vi "Initialize.vi"(8 "error in (no error)":errorcluster, 11 "DemoStepMotor in":refnum<class "DemoStepMotor.lvclass">) -> (0 "error out":errorcluster, 3 "DemoStepMotor out":refnum<class "DemoStepMotor.lvclass">)   [LabVIEW 2020, in "DemoStepMotor.lvlib" / "DemoStepMotor.lvclass"]
uses:
  DemoStepMotor.lvclass
  <vilib>/ActorFramework/Actor/Actor.lvclass
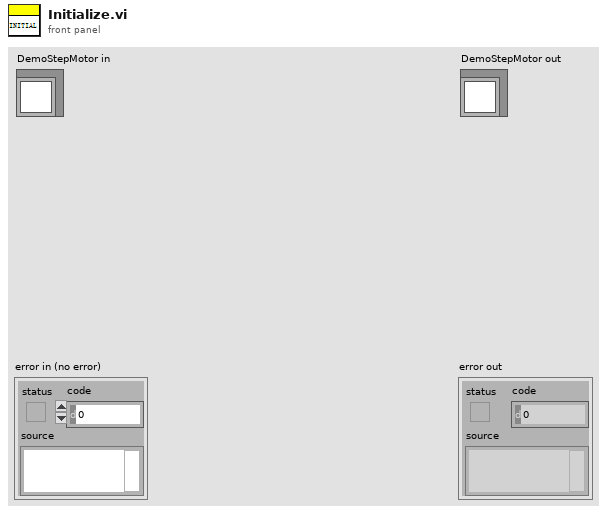
[diagram p1: front panel]
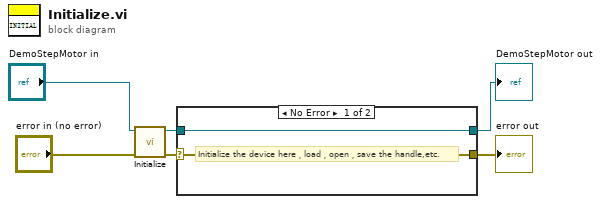
[diagram p0: block diagram]
diagram:
  n1 = call-parent "Initialize.vi"("error in (no error)"="error in (no error)", "Device in"="DemoStepMotor in") -> ("error out"=w4:errorcluster, "Device out"=w3:refnum<class "DemoStepMotor.lvclass">)  [unwired: 8 in]
  n2 = case shown="No Error" w4 {
    selector: w4 -> [w7 w10]
    tunnel: [w7 w10] -> w1
    tunnel: [w8 w9] -> w2
    tunnel: w3 -> [w8 w9]
    frame No Error {
      # "Initialize the device here，load，open，save the handle,etc."
    }
    frame Error {
    }
  }
  "error out" <- w1
  "DemoStepMotor out" <- w2
